vi "TESync Modbus Example.vi"() -> ()   [LabVIEW 2023]
uses:
  Type Definitions/Tenney Environmental Chamber Data.ctl
  Type Definitions/Tenney Chamber Status.ctl
  Type Definitions/Tenney Modbus Registers.ctl
  <vilib>/NI/Modbus Library/API/Master/Modbus Master.lvclass
panel:
  in  "Chamber Status":T1
  in  "Send Command?":bool
  in  "Update Parameters":bool
  in  "Frequency Setpoint":dbl=10.0 min=10.0 max=50.0
  in  "Humidity Setpoint":dbl min=0.0 max=100.0
  in  "Temperature Setpoint":dbl=35.0 min=35.0 max=135.0
  out "Output: Tenney Environmental Chamber Data":T2
  in  "Remote Port":u16=502
  in  "OK":bool
  in  "IP Address":string="10.2.0.248"
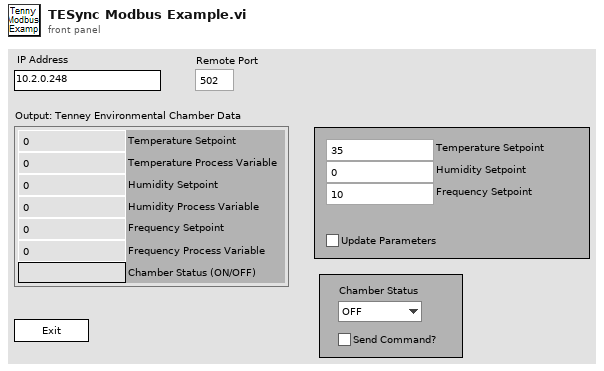
[diagram p1: front panel]
types:
  T1 = typedef "Tenney Chamber Status.ctl" = enum16{"OFF", "ON"}
  T2 = typedef "Tenney Environmental Chamber Data.ctl" = cluster{"Temperature Setpoint":dbl, "Temperature Process Variable":dbl, "Humidity Setpoint":dbl, "Humidity Process Variable":dbl, "Frequency Setpoint":dbl, "Frequency Process Variable":dbl, "Chamber Status (ON/OFF)":string}
  T3 = enum32{"Invalid", "Standard", "Closed", "Hidden", "Minimized", "Maximized"}
  T4 = enum32{"invalid app kind", "Development System", "Run Time System", "Student Edition", "Embedded LabVIEW", "Evaluation", "Custom"}
  T5 = typedef "Tenney Modbus Registers.ctl" = u16
  T6 = cluster{"Core":cluster{"Current VI Reference":refnum<vi>, "Close Panel on Exit?":bool}, "IP Address":string, "Remote Port":u16, "TCP master instance":refnum<class "Modbus Master.lvclass">, "Tenney Environmental Chamber Data":T2}
  T7 = cluster{"Current VI Reference":refnum<vi>, "Close Panel on Exit?":bool}
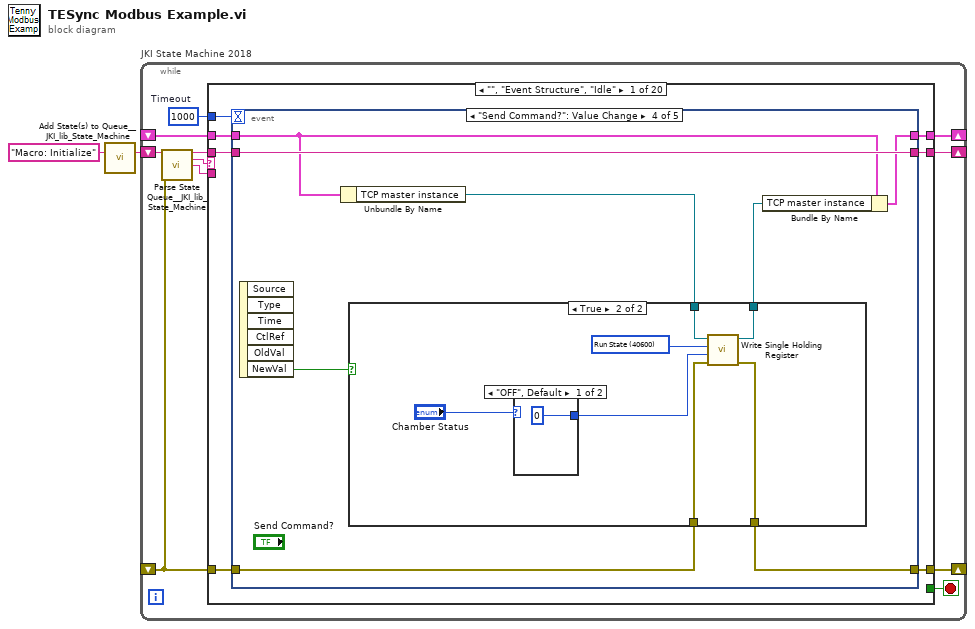
[diagram p0: block diagram]
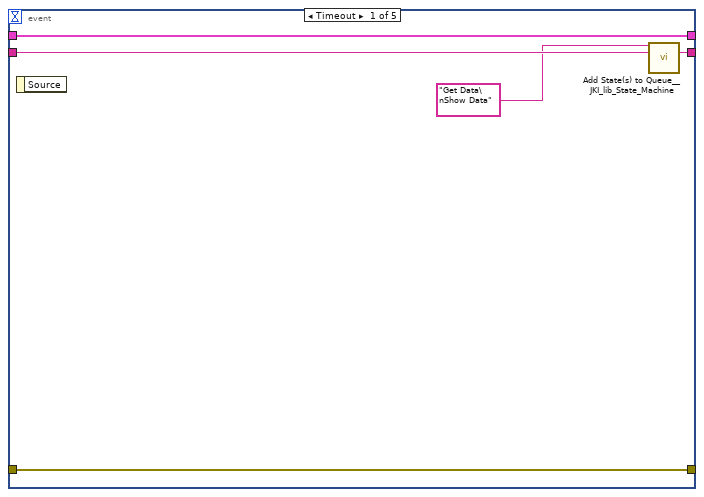
[diagram p2: hidden frame]
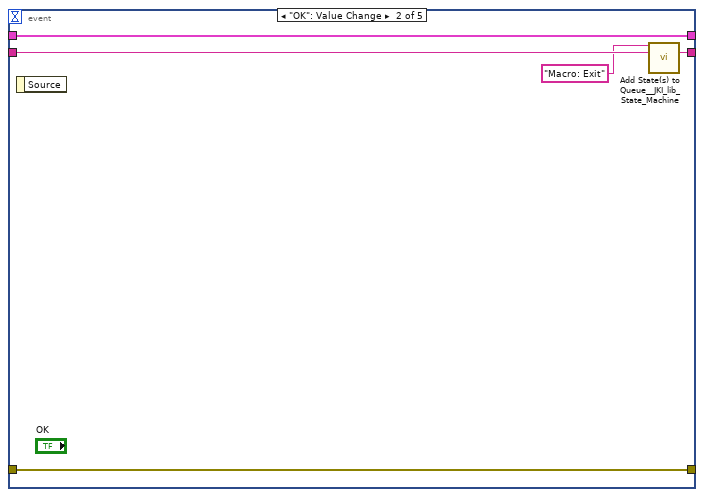
[diagram p3: hidden frame]
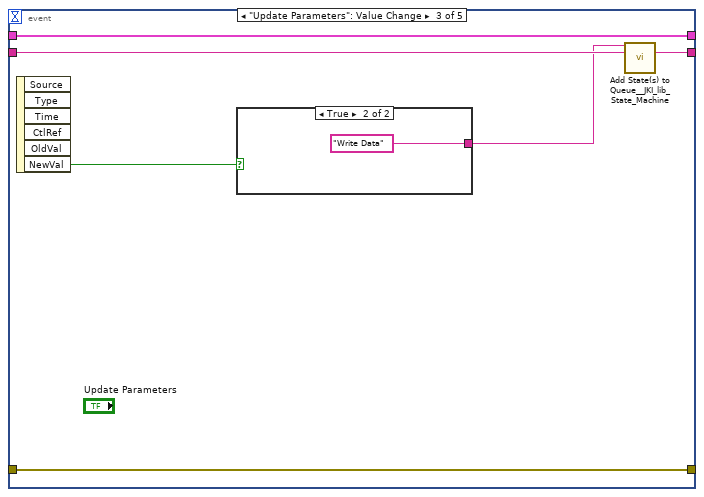
[diagram p4: hidden frame]
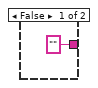
[diagram p5: hidden frame]
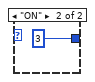
[diagram p7: hidden frame]
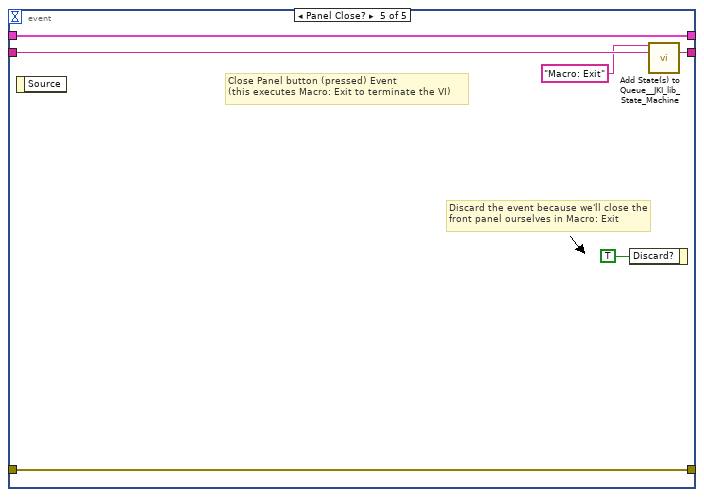
[diagram p8: hidden frame]
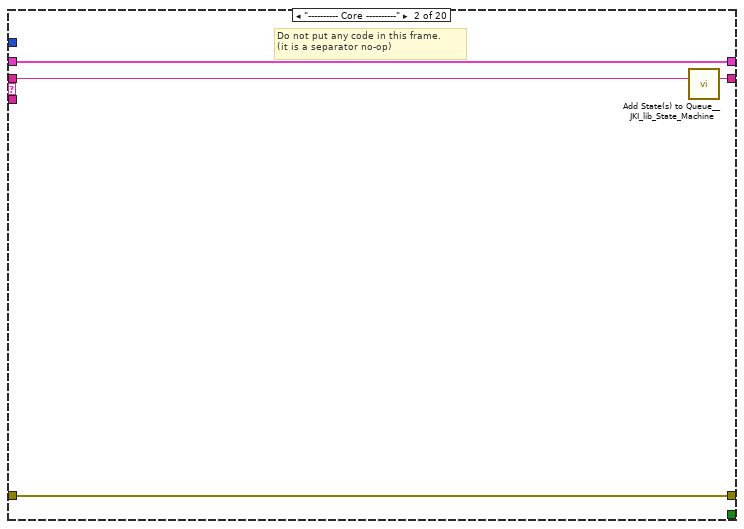
[diagram p9: hidden frame]
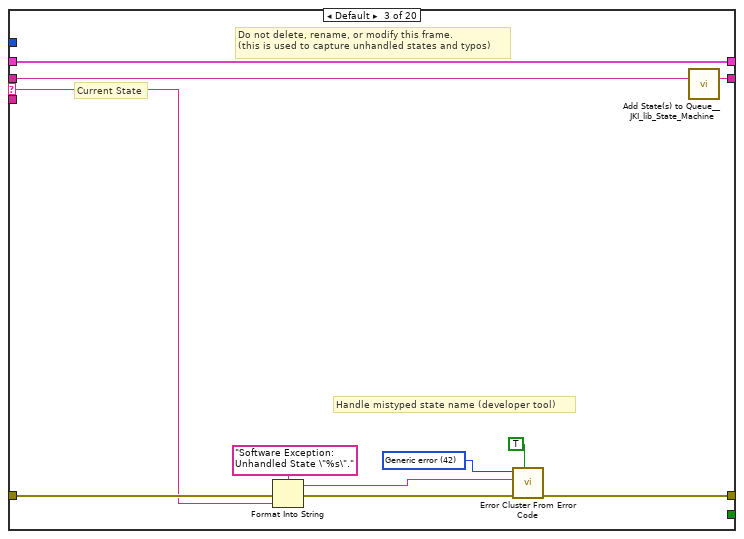
[diagram p10: hidden frame]
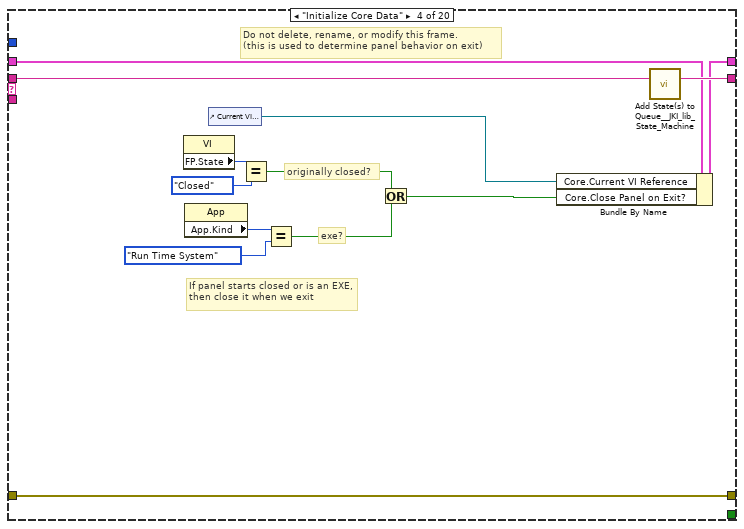
[diagram p11: hidden frame]
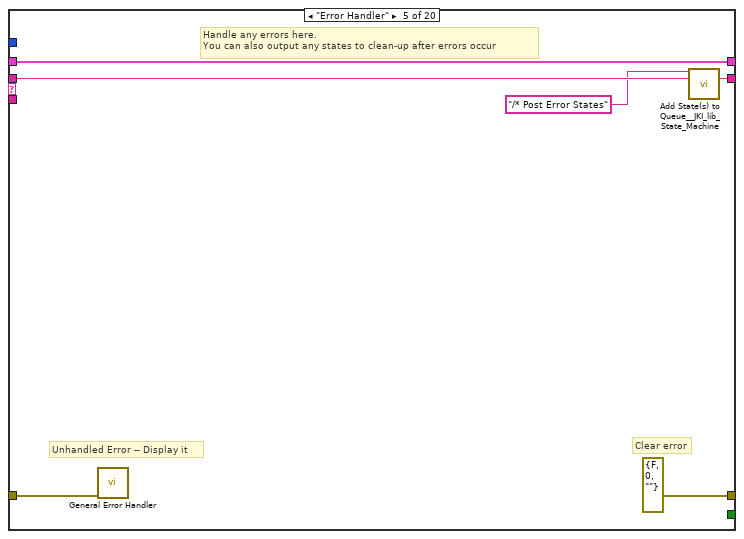
[diagram p12: hidden frame]
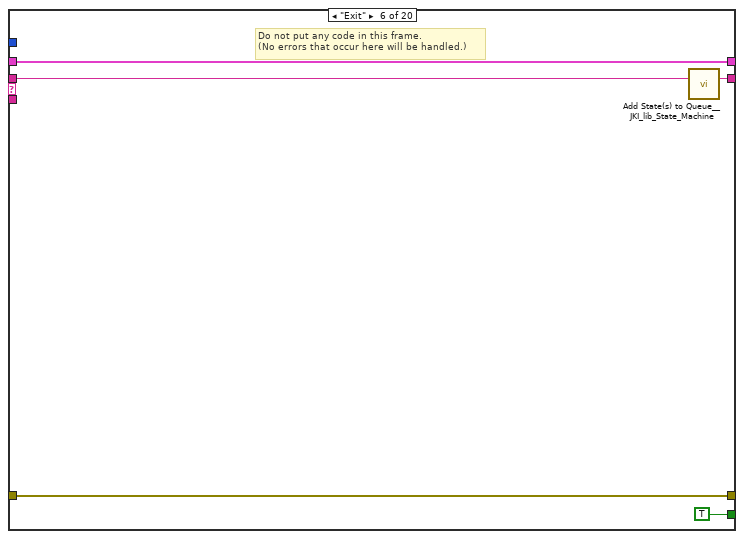
[diagram p13: hidden frame]
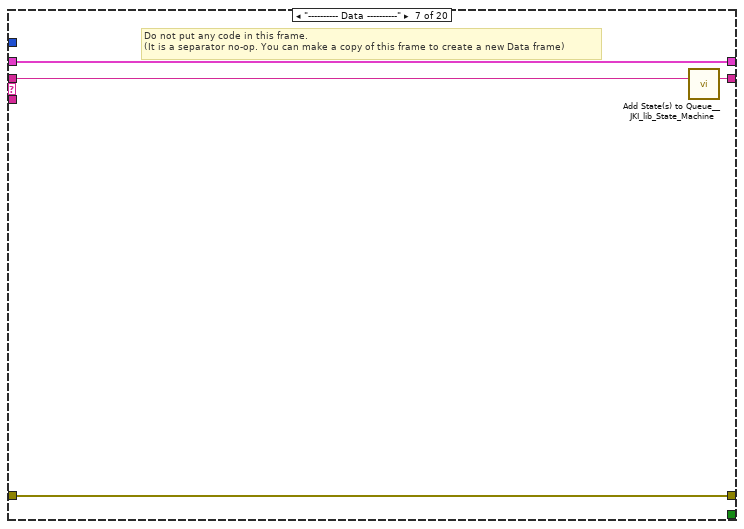
[diagram p14: hidden frame]
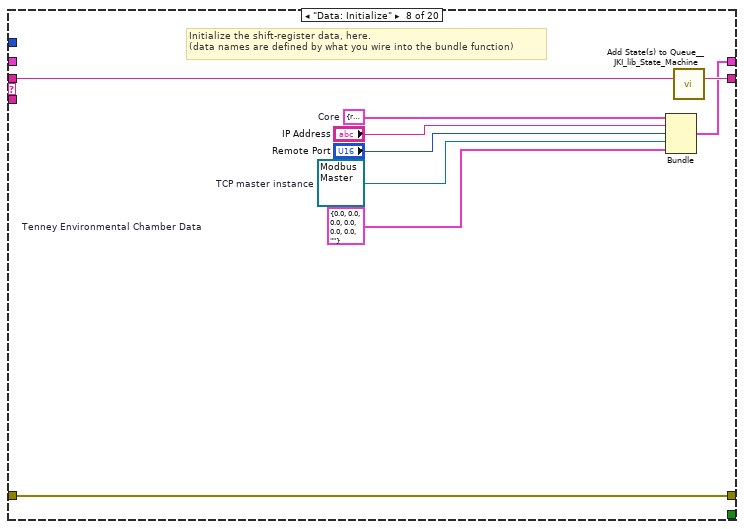
[diagram p15: hidden frame]
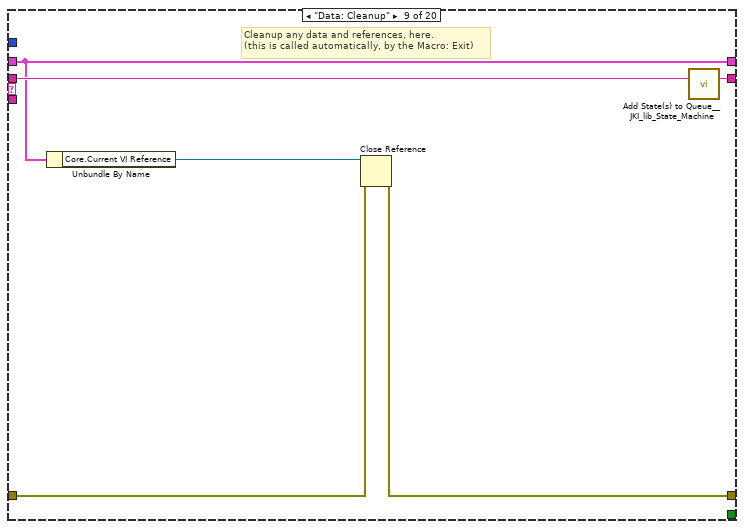
[diagram p16: hidden frame]
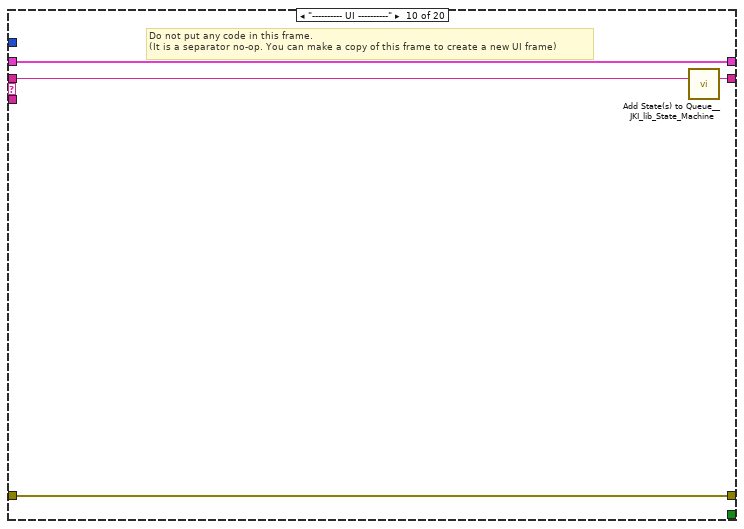
[diagram p17: hidden frame]
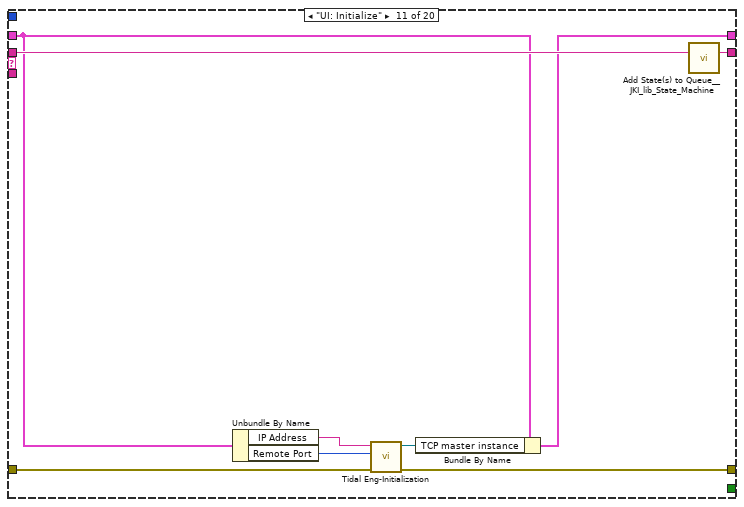
[diagram p18: hidden frame]
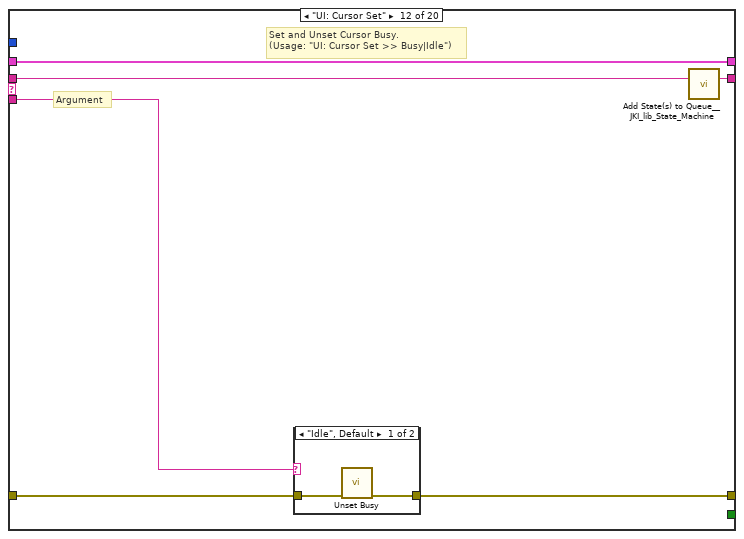
[diagram p19: hidden frame]
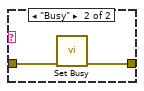
[diagram p20: hidden frame]
diagram:
  n1 = call <vilib>:"Add State(s) to Queue__JKI_lib_State_Machine.vi"("State(s) in (\"\")"="Macro: Initialize") -> ("States Out"=w2:string)  [unwired: 14 in]
  n2 = while "JKI State Machine 2018" {
    shift-right: [w6] -> _
    shift-left: _ -> [w5]
    shift-right: [w9] -> _
    shift-left: _ -> [w3]
    shift-right: [w8] -> _
    shift-left: w2 -> [w10]
    stop <- w7 stop-if-true
    w4 = 1000  # Timeout
    n3 = call <vilib>:"Parse State Queue__JKI_lib_State_Machine.vi"("State Queue"=w10, "Error In (no error)"=w3) -> ("Remaining States"=w12:string, "Current State"=w13:string, "Arguments"=w11:string)  [unwired: 11 in]
    n4 = case shown="\"\", \"Event Structure\", \"Idle\"" w13 {
      selector: w13 -> [_ _ w68 _ _ _ _ _ _ _ _ _ _ _ _ _ _ _ _ _]
      tunnel: w12 -> [w20 w67 w72 w91 w97 w102 w106 w115 w121 w125 w134 w140 w151 w220 w225 w237 w241 w250 w265 w270]
      tunnel: w11 -> [_ _ _ _ _ _ _ _ _ _ _ w135 w145 _ _ _ _ _ _ _]
      tunnel: w5 -> [w18 w64 w70 w84 w94 w100 w103 _ w116 w122 w128 w138 w147 w217 w222 w235 w238 w245 w262 w267]
      tunnel: [w17 w65 w74 w88 errorcluster {"status"=FALSE, "code"=0, "source"=""} ("error out") w99 w104 w112 w117 w123 w131 w136 w148 w218 w223 w227 w239 w247 w257 w268] -> w9
      tunnel: w3 -> [w16 w65 w73 w88 w93 w99 w104 w112 w118 w123 w132 w137 w149 w218 w223 w228 w239 w248 w260 w268]
      tunnel: [w19 w66 w71 w90 w96 w101 w105 w114 w120 w124 w133 w139 w150 w219 w224 w236 w240 w249 w264 w269] -> w8
      tunnel: [_ _ _ _ _ TRUE _ _ _ _ _ _ _ _ _ _ _ _ _ _] -> w7
      tunnel: [w15 w64 w70 w89 w94 w100 w103 w113 w116 w122 w127 w138 w147 w217 w222 w235 w238 w244 w261 w267] -> w6
      tunnel: w4 -> [w14 _ _ _ _ _ _ _ _ _ _ _ _ _ _ _ _ _ _ _]
      frame "", "Event Structure", "Idle" {
        n5 = event shown="[3] \"Send Command?\": Value Change" {
          selector: _ -> [_ _ _ _ _]
          dyn-events: _ -> [_ _ _ _ _]
          timeout: w14 -> [_ _ _ _ _]
          tunnel: w20 -> [w25 w30 w34 w46 w63]
          tunnel: [w24 w29 w33 w46 w62] -> w19
          tunnel: w18 -> [w22 w27 w35 w42 w60]
          tunnel: [w23 w28 w36 w44 w61] -> w17
          tunnel: w16 -> [w23 w28 w36 w45 w61]
          tunnel: [w22 w27 w35 w41 w60] -> w15
          event Timeout {
            n6 = event-data() -> ()  [unwired: 1 in, 1 out]
            n7 = call <vilib>:"Add State(s) to Queue__JKI_lib_State_Machine.vi"("State(s) in Front (\"\")"="Get Data\nShow Data" ("State(s) in Front (\"\")"), "State(s) in (\"\")"=w25) -> ("States Out"=w24:string)  [unwired: 13 in]
          }
          event "OK": Value Change {
            n8 = event-data() -> ()  [unwired: 1 in, 1 out]
            n9 = call <vilib>:"Add State(s) to Queue__JKI_lib_State_Machine.vi"("State(s) in Front (\"\")"="Macro: Exit", "State(s) in (\"\")"=w30) -> ("States Out"=w29:string)  [unwired: 13 in]
          }
          event "Update Parameters": Value Change {
            n10 = event-data() -> ("NewVal"=w31:bool)  [unwired: 1 in, 5 out]
            n11 = case shown="True" w31 {
              tunnel: ["" "Write Data"] -> w32
              frame False {
              }
              frame True {
              }
            }
            n12 = call <vilib>:"Add State(s) to Queue__JKI_lib_State_Machine.vi"("State(s) in Front (\"\")"=w32, "State(s) in (\"\")"=w34) -> ("States Out"=w33:string)  [unwired: 13 in]
          }
          event "Send Command?": Value Change {
            n13 = event-data() -> ("NewVal"=w39:bool)  [unwired: 1 in, 5 out]
            n14 = Unbundle By Name(w42) -> ("TCP master instance"=w43:refnum<class "Modbus Master.lvclass">)
            n15 = case shown="True" w39 {
              tunnel: w45 -> [w47 w55]
              tunnel: [w47 w54] -> w44
              tunnel: w43 -> [w48 w53]
              tunnel: [w48 w51] -> w40
              frame False {
              }
              frame True {
                w52 = T5 40600 items=["Ch1 Setpoint"=40100, "Ch1 Process Variable"=40103, "Ch2 Setpoint"=40200, "Ch2 Process Variable"=40203, "Ch3 Setpoint"=40300, "Ch3 Process Variable"=40303, "All Events Mask"=40500, "Run State"=40600] ("Modbus Registers")
                n16 = case shown="\"OFF\", Default" "Chamber Status" {
                  tunnel: [u16 0 ("register to write") u16 3 ("register to write")] -> w49
                  frame "OFF", Default {
                  }
                  frame "ON" {
                  }
                }
                n17 = call-dynamic "Write Single Holding Register.vi"("error in"=w55, "register to write"=w49, "address"=w52, "Modbus master in"=w53) -> ("error out"=w54:errorcluster, "Modbus master out"=w51:refnum<class "Modbus Master.lvclass">)  [unwired: 6 in]
              }
            }
            n18 = Bundle By Name(cluster=w42, "TCP master instance"=w40) -> (w41:T6)
          }
          event Panel Close? {
            # "Discard the event because we'll close the front panel ourselves in Macro: Exit"
            # "Close Panel button (pressed) Event\n(this executes Macro: Exit to terminate the VI)"
            n19 = event-data() -> ()  [unwired: 1 in, 1 out]
            n20 = event-data("Discard?"=TRUE) -> ()  [unwired: 1 in, 1 out]
            n21 = call <vilib>:"Add State(s) to Queue__JKI_lib_State_Machine.vi"("State(s) in Front (\"\")"="Macro: Exit", "State(s) in (\"\")"=w63) -> ("States Out"=w62:string)  [unwired: 13 in]
          }
        }
      }
      frame "---------- Core ----------" {
        # "Do not put any code in this frame.\n(it is a separator no-op)"
        n22 = call <vilib>:"Add State(s) to Queue__JKI_lib_State_Machine.vi"("State(s) in (\"\")"=w67) -> ("States Out"=w66:string)  [unwired: 14 in]
      }
      frame Default {
        w77 = 42 items=["No error", "Argument error", "Memory is full", "Out of zone", "End of file", "File already open", "Generic file I/O error", "File not found", "File permission error", "Disk is full", "Duplicate path", "Too many files open", "System feature not enabled", "Resource file not found", "Cannot add resource", "Resource not found", "Image not found", "Image memory error", "Pen does not exist", "Config type invalid", "Config token not found", "Config parse error", "Config memory error", "Bad external code format", "Bad external code offset", "External code not present", "Null window", "Destroy window error", "Null menu", "Print aborted", "Bad print record", "Print driver error", "Windows error during printing", "Memory error during printing", "Print dialog error", "Generic print error", "Invalid device refnum", "Device not found", "Device parameter error", "Device unit error", "Cannot open device", "Device call aborted", "Generic error", "Cancelled by user", "Object ID too low", "Object ID too high", "Object not in heap", "Unknown heap", "Unknown object (invalid DefProc)", "Unknown object (DefProc not in table)", "Message out of range", "Invalid (null) method", "Unknown message", "Manager call not supported", "Bad address", "Network operation in progress", "Network operation timed out", "Connection is busy", "Network attribute not supported", "Network error", "Address in use", "System out of memory", "Connection aborted", "Connection refused", "Not connected", "Already connected", "Connection closed", "Initialization error (interapplication manager)", "Bad occurrence", "Wait on unbound occurrence handler", "Occurrence queue overflow", "Datalog type conflict", "Unused", "Unrecognized type (interapplication manager)", "Memory corrupt", "Failed to make temporary DLL", "Old CIN version", "Drag socket not found", "Failed to load drop-object", "Failed to register OLE object", "Failed to release OLE object", "Format specifier type mismatch", "Unknown format specifier", "Too few format specifiers", "Too many format specifiers", "Scan failed", "Newer CIN version", "Error converting to variant", "Runtime menu error", "Password tampered", "Variant attribute not found", "Incompatible variant data type", "Event data is not available", "Event Store is not present", "Occurrence is not found", "Event Queue is not created", "Event info is not available", "Refnum passed is NULL", "Error retrieving Class GUID", "Error retrieving CoClass GUID", "Error retrieving TypeLib GUID.", "Bad built application magic bytes.", "Specific driver is different from the specific driver associated with the Logical Name.", "There is no session opened to the class driver.", "Max Error", "MAX - Error with config objects", "MAX - Error loading configuration", "MAX - Group not supported"]
        # "Current State"
        # "Do not delete, rename, or modify this frame.\n(this is used to capture unhandled states and typos)"
        # "Handle mistyped state name (developer tool)"
        n23 = Format Into String(format string="Software Exception: Unhandled State \"%s\"." ("message"), error in=w73, w68) -> (resulting string=w76:string, error out=w75:errorcluster)  [unwired: 1 in]
        n24 = call <vilib>:"Error Cluster From Error Code.vi"("show call chain? (False)"=TRUE, "error in (no error)"=w75, "error message (\"\")"=w76, "error code (0)"=w77) -> ("error out"=w74:errorcluster)  [unwired: 5 in]
        n25 = call <vilib>:"Add State(s) to Queue__JKI_lib_State_Machine.vi"("State(s) in (\"\")"=w72) -> ("States Out"=w71:string)  [unwired: 14 in]
      }
      frame "Initialize Core Data" {
        # "Do not delete, rename, or modify this frame.\n(this is used to determine panel behavior on exit)"
        # "originally closed?"
        # "exe?"
        # "If panel starts closed or is an EXE, then close it when we exit"
        n26 = property class="VI"() -> ("FP.State"=w81:T3)  [unwired: 2 in, 2 out]
        n27 = property class="App"() -> ("App.Kind"=w87:T4)  [unwired: 2 in, 2 out]
        n28 = control-ref of="Current VI Reference"() -> (w82:refnum<vi>)
        n29 = Equal?(x=w81, y=T3."Closed" ("Front Panel Window:State")) -> (x = y?=w79:bool)
        n30 = Equal?(x=w87, y=T4."Run Time System" ("Application:Kind")) -> (x = y?=w85:bool)
        n31 = Or(x=w79, y=w85) -> (x .or. y?=w83:bool)
        n32 = Bundle By Name(cluster=w84, "Core.Current VI Reference"=w82, "Core.Close Panel on Exit?"=w83) -> (w89:T6)
        n33 = call <vilib>:"Add State(s) to Queue__JKI_lib_State_Machine.vi"("State(s) in (\"\")"=w91) -> ("States Out"=w90:string)  [unwired: 14 in]
      }
      frame "Error Handler" {
        # "Unhandled Error -- Display it"
        # "Handle any errors here.\nYou can also output any states to clean-up after errors occur"
        # "Clear error"
        n34 = call <vilib>:"General Error Handler.vi"("error in (no error)"=w93) -> ()  [unwired: 10 in, 5 out]
        n35 = call <vilib>:"Add State(s) to Queue__JKI_lib_State_Machine.vi"("State(s) in Front (\"\")"="/* Post Error States", "State(s) in (\"\")"=w97) -> ("States Out"=w96:string)  [unwired: 13 in]
      }
      frame "Exit" {
        # "Do not put any code in this frame.\n(No errors that occur here will be handled.)"
        n36 = call <vilib>:"Add State(s) to Queue__JKI_lib_State_Machine.vi"("State(s) in (\"\")"=w102) -> ("States Out"=w101:string)  [unwired: 14 in]
      }
      frame "---------- Data ----------" {
        # "Do not put any code in this frame.\n(It is a separator no-op. You can make a copy of this frame to create a new Data frame)"
        n37 = call <vilib>:"Add State(s) to Queue__JKI_lib_State_Machine.vi"("State(s) in (\"\")"=w106) -> ("States Out"=w105:string)  [unwired: 14 in]
      }
      frame "Data: Initialize" {
        w107 = T2 {"Temperature Setpoint"=0.0, "Temperature Process Variable"=0.0, "Humidity Setpoint"=0.0, "Humidity Process Variable"=0.0, "Frequency Setpoint"=0.0, "Frequency Process Variable"=0.0, "Chamber Status (ON/OFF)"=""}  # Tenney Environmental Chamber Data
        w108 = refnum<class "Modbus Master.lvclass"> refnum  # TCP master instance
        w111 = T7 {"Current VI Reference"=refnum, "Close Panel on Exit?"=FALSE}  # Core
        # "Initialize the shift-register data, here.\n(data names are defined by what you wire into the bundle function)"
        n38 = Bundle("Core"=w111, "IP Address"="IP Address", "Remote Port"="Remote Port", "TCP master instance"=w108, "Tenney Environmental Chamber Data"=w107) -> (w113:T6)  [unwired: 1 in]
        n39 = call <vilib>:"Add State(s) to Queue__JKI_lib_State_Machine.vi"("State(s) in (\"\")"=w115) -> ("States Out"=w114:string)  [unwired: 14 in]
      }
      frame "Data: Cleanup" {
        # "Cleanup any data and references, here.\n(this is called automatically, by the Macro: Exit)"
        n40 = Unbundle By Name(w116) -> ("Core.Current VI Reference"=w119:refnum<vi>)
        n41 = Close Reference(reference=w119, error in (no error)=w118) -> (error out=w117:errorcluster)
        n42 = call <vilib>:"Add State(s) to Queue__JKI_lib_State_Machine.vi"("State(s) in (\"\")"=w121) -> ("States Out"=w120:string)  [unwired: 14 in]
      }
      frame "---------- UI ----------" {
        # "Do not put any code in this frame.\n(It is a separator no-op. You can make a copy of this frame to create a new UI frame)"
        n43 = call <vilib>:"Add State(s) to Queue__JKI_lib_State_Machine.vi"("State(s) in (\"\")"=w125) -> ("States Out"=w124:string)  [unwired: 14 in]
      }
      frame "UI: Initialize" {
        n44 = Unbundle By Name(w128) -> ("IP Address"=w130:string, "Remote Port"=w129:u16)
        n45 = call "Tidal Eng-Initialization.vi"("error in (no error)"=w132, "Remote Port"=w129, "IP Address"=w130) -> ("error out"=w131:errorcluster, "Modbus Master out"=w126:refnum<class "Modbus Master.lvclass">)  [unwired: 7 in]
        n46 = Bundle By Name(cluster=w128, "TCP master instance"=w126) -> (w127:T6)
        n47 = call <vilib>:"Add State(s) to Queue__JKI_lib_State_Machine.vi"("State(s) in (\"\")"=w134) -> ("States Out"=w133:string)  [unwired: 14 in]
      }
      frame "UI: Cursor Set" {
        # "Argument"
        # "Set and Unset Cursor Busy.\n(Usage: \"UI: Cursor Set >> Busy|Idle\")"
        n48 = case shown="\"Idle\", Default" w135 {
          tunnel: w137 -> [w142 w144]
          tunnel: [w141 w143] -> w136
          frame "Idle", Default {
            n49 = call <vilib>:"Unset Busy.vi"("error in (no error)"=w142) -> ("error out"=w141:errorcluster)  [unwired: 10 in]
          }
          frame "Busy" {
            n50 = call <vilib>:"Set Busy.vi"("error in (no error)"=w144) -> ("error out"=w143:errorcluster)  [unwired: 9 in, 1 out]
          }
        }
        n51 = call <vilib>:"Add State(s) to Queue__JKI_lib_State_Machine.vi"("State(s) in (\"\")"=w140) -> ("States Out"=w139:string)  [unwired: 14 in]
      }
      frame "UI: Front Panel State" {
        # "Argument"
        # "Set Front Panel Open or Closed\n(Usage: \"UI: Front Panel State >> Open|Close\")"
        n52 = Unbundle By Name(w147) -> ("Core.Current VI Reference"=w146:refnum<vi>)
        n53 = case shown="\"Minimize\", \"Minimized\"" w145 {
          tunnel: w149 -> [w157 w172 w183 w196 w209]
          tunnel: [w159 w173 w185 w198 w211] -> w148
          tunnel: w146 -> [w158 w170 w184 w197 w210]
          frame "Open", "Standard", Default {
            w152 = T3."Standard" ("State")
            n54 = property class="VI"(reference=w158, error in=w157) -> (reference out=w155:refnum<vi>, error out=w156:errorcluster, "FP.State"=w154:T3)
            n55 = Not Equal?(x=w154, y=w152) -> (x != y?=w153:bool)
            n56 = case shown="True" w153 {
              tunnel: [w163 w165] -> w159
              tunnel: w156 -> [w162 w165]
              tunnel: w155 -> [w161 _]
              tunnel: w152 -> [w160 _]
              frame True {
                n57 = invoke class="VI" method="FP.Open"(reference=w161, error in=w162, "Activate"=TRUE, "State"=w160) -> (error out=w163:errorcluster)  [unwired: 1 in, 4 out]
              }
              frame False {
              }
            }
          }
          frame "Close", "Closed" {
            n58 = property class="VI"(reference=w170, error in=w172) -> (reference out=w169:refnum<vi>, error out=w171:errorcluster, "FP.State"=w167:T3)
            n59 = Not Equal?(x=w167, y=T3."Closed" ("Front Panel Window:State")) -> (x != y?=w166:bool)
            n60 = case shown="True" w166 {
              tunnel: [w174 w177] -> w173
              tunnel: w171 -> [w174 w176]
              tunnel: w169 -> [_ w175]
              frame False {
              }
              frame True {
                n61 = invoke class="VI" method="FP.Close"(reference=w175, error in=w176) -> (error out=w177:errorcluster)  [unwired: 1 in, 2 out]
              }
            }
          }
          frame "Hidden", "Hide" {
            w178 = T3."Hidden" ("State")
            n62 = property class="VI"(reference=w184, error in=w183) -> (reference out=w181:refnum<vi>, error out=w182:errorcluster, "FP.State"=w180:T3)
            n63 = Not Equal?(x=w180, y=w178) -> (x != y?=w179:bool)
            n64 = case shown="True" w179 {
              tunnel: [w189 w190] -> w185
              tunnel: w182 -> [w188 w190]
              tunnel: w181 -> [w187 _]
              tunnel: w178 -> [w186 _]
              frame True {
                n65 = invoke class="VI" method="FP.Open"(reference=w187, error in=w188, "State"=w186) -> (error out=w189:errorcluster)  [unwired: 2 in, 4 out]
              }
              frame False {
              }
            }
          }
          frame "Minimize", "Minimized" {
            w191 = T3."Minimized" ("State")
            n66 = property class="VI"(reference=w197, error in=w196) -> (reference out=w194:refnum<vi>, error out=w195:errorcluster, "FP.State"=w193:T3)
            n67 = Not Equal?(x=w193, y=w191) -> (x != y?=w192:bool)
            n68 = case shown="True" w192 {
              tunnel: [w202 w203] -> w198
              tunnel: w195 -> [w201 w203]
              tunnel: w194 -> [w200 _]
              tunnel: w191 -> [w199 _]
              frame True {
                n69 = invoke class="VI" method="FP.Open"(reference=w200, error in=w201, "State"=w199) -> (error out=w202:errorcluster)  [unwired: 2 in, 4 out]
              }
              frame False {
              }
            }
          }
          frame "Maximize", "Maximized" {
            w204 = T3."Maximized" ("State")
            n70 = property class="VI"(reference=w210, error in=w209) -> (reference out=w207:refnum<vi>, error out=w208:errorcluster, "FP.State"=w206:T3)
            n71 = Not Equal?(x=w206, y=w204) -> (x != y?=w205:bool)
            n72 = case shown="True" w205 {
              tunnel: [w215 w216] -> w211
              tunnel: w208 -> [w214 w216]
              tunnel: w207 -> [w213 _]
              tunnel: w204 -> [w212 _]
              frame True {
                n73 = invoke class="VI" method="FP.Open"(reference=w213, error in=w214, "State"=w212) -> (error out=w215:errorcluster)  [unwired: 2 in, 4 out]
              }
              frame False {
              }
            }
          }
        }
        n74 = call <vilib>:"Add State(s) to Queue__JKI_lib_State_Machine.vi"("State(s) in (\"\")"=w151) -> ("States Out"=w150:string)  [unwired: 14 in]
      }
      frame "---------- Macro ----------" {
        # "Do not put any code in this frame.\n(It is a separator no-op. You can make a copy of this frame to create a new Macro frame)"
        n75 = call <vilib>:"Add State(s) to Queue__JKI_lib_State_Machine.vi"("State(s) in (\"\")"=w220) -> ("States Out"=w219:string)  [unwired: 14 in]
      }
      frame "Macro: Initialize" {
        w221 = "Data: Initialize\nInitialize Core Data\nUI: Initialize\nUI: Front Panel State >> Open"  # Data: Initialize Initialize Core Data UI: Initialize UI: Front Panel State >> Open
        # "Initialization Macro\n(This is called once, when the VI starts)"
        n76 = call <vilib>:"Add State(s) to Queue__JKI_lib_State_Machine.vi"("State(s) in Front (\"\")"=w221, "State(s) in (\"\")"=w225) -> ("States Out"=w224:string)  [unwired: 13 in]
      }
      frame "Macro: Exit" {
        # "Exit Macro\n(This is called once, when the VI exits)"
        n77 = Unbundle By Name(w235) -> ("Core.Close Panel on Exit?"=w234:bool, "TCP master instance"=w226:refnum<class "Modbus Master.lvclass">)
        n78 = Select(t="UI: Front Panel State >> Close", s=w234, f="") -> (s? t:f=w231:string)
        n79 = call <vilib>:"Add State(s) to Queue__JKI_lib_State_Machine.vi"("State(s) in (\"\")"=w231, "State(s) at Back (\"\")"="Data: Cleanup\nExit") -> ("States Out"=w229:string)  [unwired: 13 in]
        n80 = call-dynamic "Shutdown.vi"("error in"=w228, "Modbus master in"=w226) -> ("error out"=w227:errorcluster)  [unwired: 9 in]
        n81 = call <vilib>:"Add State(s) to Queue__JKI_lib_State_Machine.vi"("State(s) in Front (\"\")"=w229, "State(s) in (\"\")"=w237) -> ("States Out"=w236:string)  [unwired: 13 in]
      }
      frame "---------- New Category ----------" {
        # "Template Separator\n(You can make a copy of, or modify, this frame)"
        n82 = call <vilib>:"Add State(s) to Queue__JKI_lib_State_Machine.vi"("State(s) in (\"\")"=w241) -> ("States Out"=w240:string)  [unwired: 14 in]
      }
      frame "Get Data" {
        n83 = Unbundle By Name(w245) -> ("TCP master instance"=w246:refnum<class "Modbus Master.lvclass">)
        n84 = call "Tidal Eng-Modbus Data.vi"("error in (no error)"=w248, "Modbus master in"=w246) -> ("error out"=w247:errorcluster, "Tenney Environmental Chamber Data Output"=w242:T2, "Modbus master out"=w243:refnum<class "Modbus Master.lvclass">)  [unwired: 6 in, 1 out]
        n85 = Bundle By Name(cluster=w245, "TCP master instance"=w243, "Tenney Environmental Chamber Data"=w242) -> (w244:T6)
        n86 = call <vilib>:"Add State(s) to Queue__JKI_lib_State_Machine.vi"("State(s) in (\"\")"=w250) -> ("States Out"=w249:string)  [unwired: 14 in]
      }
      frame "Write Data" {
        n87 = Unbundle By Name(w262) -> ("TCP master instance"=w263:refnum<class "Modbus Master.lvclass">)
        n88 = call "Tidal Eng-Write Temperature Setpoint.vi"("error in (no error)"=w260, "Temperature (°F)"="Temperature Setpoint", "Modbus master in"=w263) -> ("error out"=w259:errorcluster, "Modbus master out"=w254:refnum<class "Modbus Master.lvclass">)  [unwired: 7 in]
        n89 = call "Tidal Eng-Write Humidity Setpoint.vi"("error in (no error)"=w259, "Humidity (%)"="Humidity Setpoint", "Modbus master in"=w254) -> ("error out"=w258:errorcluster, "Modbus master out"=w255:refnum<class "Modbus Master.lvclass">)  [unwired: 7 in]
        n90 = call "Tidal Eng-Write Frequency Setpoint.vi"("error in (no error)"=w258, "Frequency (Hz)"="Frequency Setpoint", "Modbus master in"=w255) -> ("error out"=w257:errorcluster, "Modbus master out"=w256:refnum<class "Modbus Master.lvclass">)  [unwired: 7 in]
        n91 = Bundle By Name(cluster=w262, "TCP master instance"=w256) -> (w261:T6)
        n92 = call <vilib>:"Add State(s) to Queue__JKI_lib_State_Machine.vi"("State(s) in (\"\")"=w265) -> ("States Out"=w264:string)  [unwired: 14 in]
      }
      frame "Show Data" {
        n93 = Unbundle By Name(w267) -> ("Tenney Environmental Chamber Data"=→"Output: Tenney Environmental Chamber Data":T2)
        n94 = call <vilib>:"Add State(s) to Queue__JKI_lib_State_Machine.vi"("State(s) in (\"\")"=w270) -> ("States Out"=w269:string)  [unwired: 14 in]
      }
    }
  }
